vi "ExtractIntegerFromString.vi"(10 "String":string) -> (2 "number":i32)   [LabVIEW 2020]
uses:
  Match Regular Expression.xnode
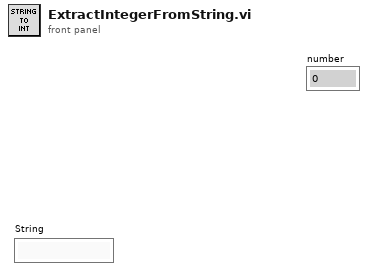
[diagram p1: front panel]
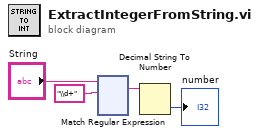
[diagram p0: block diagram]
diagram:
  n1 = xnode "Match Regular Expression"("input string"="String", "regular expression"="\\d+") -> ("whole match"=w2:string)  [unwired: 4 in, 4 out]
  n2 = Decimal String To Number(string=w2) -> (number=→"number":i32)  [unwired: 2 in, 1 out]
